vi "Test Parameter Globals_1.0.0.vi"() -> ()   [LabVIEW 2018]
panel:
  out "Global_Pass(T)":bool
  out "LOT ID":string
  out "EMP Name":string
  out "OperatorInfo":string
  out "BarCodeInfo":string
  out "Setup.vi Error":errorcluster
  in  "Use TAIL":bool caption="Place entry into test log"
  out "Parameter                                Result":string[][](array[string])
  out "Payload Results":string[](array[string])
  out "Loop Names":string[](array[string])=["TEMP", "VCC", "GAIN"]
  in  "Show Close FP":bool=TRUE
  in  "Run Close vi":bool=TRUE
  in  "Show Setup FP":bool=TRUE
  in  "Close vi":path=path "C:/IdtATE/Charactorization Tests/F1200/Linearity/F1200_Linearity_Setup_0.0.0.1.vi"
  out "Global SN":string
  out "Loop Info":string[](array[string])
  out "Total Test Time":string="1.000"
  out "Seq End Time":string="2/16/2011 9:37 AM"
  out "Seq Start Time":string="2/16/2011 9:36 AM"
  in  "User Prompt for SN (T)":bool
  out "Test Name":string
  in  "Test Parameters File":path
  out "Computer Name":string
  in  "Show Payload FP":bool=TRUE
  out "Input Constants Name Out":string[](array[string])=["Pout Ref", "Fdelta", "FSIQ Analyzer Atten Value", "FSIQ Ref Lvl Offset", "FSIQ Trace B RBW", "PS1-1 Current Limit"]
  out "Column Headers Global":string[](array[string])
  in  "Run Payload vi":bool=TRUE
  in  "Run Setup vi":bool=TRUE
  out "Input Constants Out":string[](array[string])=["3", "1000000"]
  in  "Setup Path":path=path "C:/IdtATE/Charactorization Tests/F1200/Linearity/F1200_Linearity_Setup_0.0.0.1.vi"
  in  "Payload Path":path=path "C:/IdtATE/Charactorization Tests/F1200/Linearity/F1200_Linearity_Payload_0.0.0.1.vi"
  out "# of iterations":i32=3
  out "Test Parameters":string[][](array[string])=[["4.750000", "100000000.000000", "", "", "", ""], ["5.000000", "100000000.000000", "", "", "", ""], ["5.250000", "100000000.000000", "", "", "", ""]]
  # "Information Fron Sequencer"
  # "Information From Test Parameters (Get Loop Parameters)"
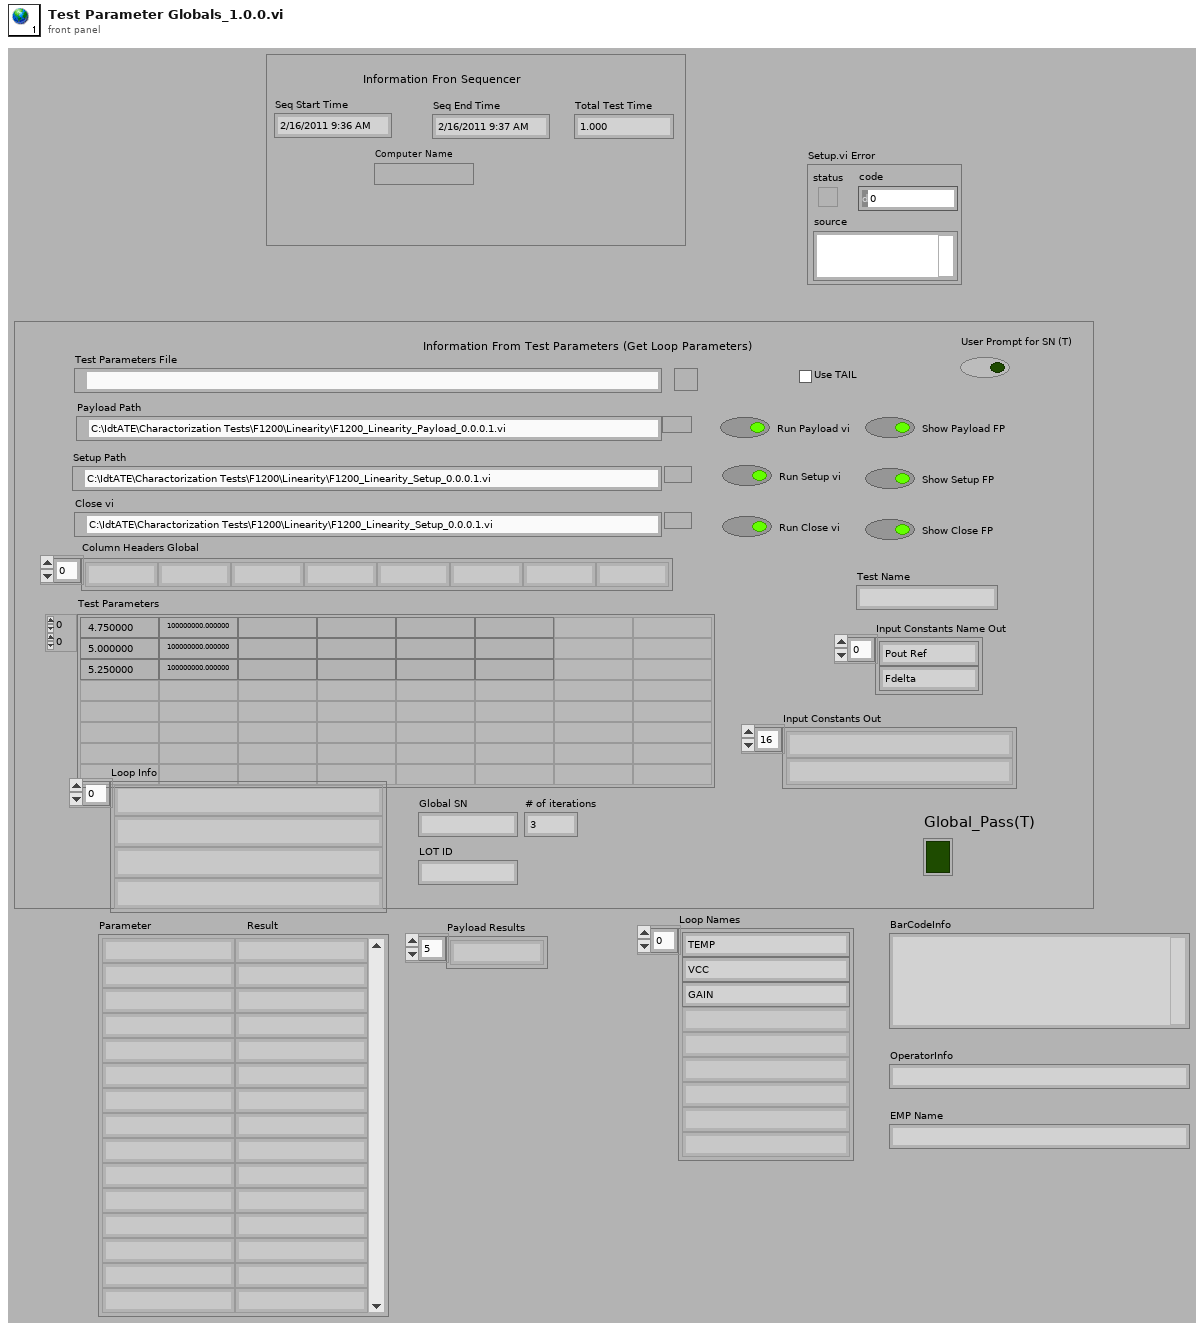
[diagram p1: front panel]
diagram:
